vi "GEOM_AdjustDetStruct.vi"(7 "corr unbin":bool, 9 "GEOM_CorrectedFPA in":T1[](array[typedef]), 10 "GEOM_FPAReadModes":T2[](array[typedef]) {"Amplifiers"."fliped" items=["none", "horizontal", "vertical"]; "Amplifiers"."type" items=["LL", "LR", "UL", "UR"]}) -> ()   [LabVIEW 2016]
uses:
  GEOM_FPAReadMode.ctl
  GEOM_Amplifier.ctl
  GEOM_AmpType.ctl
  GEOM_ROI.ctl
  GEOM_Coords.ctl
  GEOM_CorrectedFPA.ctl
  GEOM_VAR_action.ctl
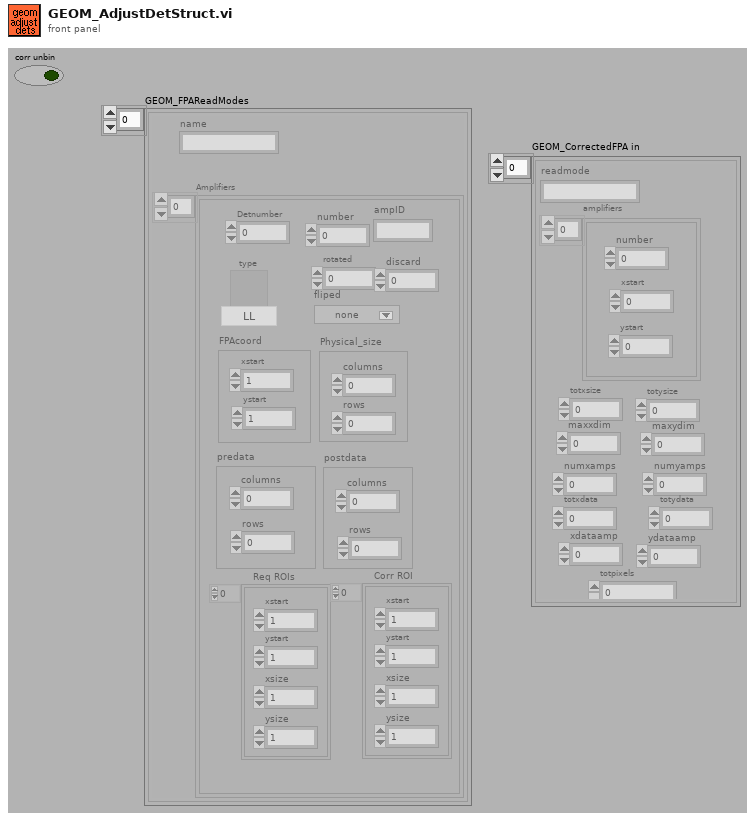
[diagram p1: front panel]
types:
  T1 = typedef "GEOM_CorrectedFPA.ctl" = cluster{"readmode":string, "amplifiers":cluster{"number":i32, "xstart":i32, "ystart":i32}[], "totxsize":i32, "totysize":i32, "maxxdim":i32, "maxydim":i32, "numxamps":i32, "numyamps":i32, "totxdata":i32, "totydata":i32, "xdataamp":i32, "ydataamp":i32, "totpixels":i32}
  T2 = typedef "GEOM_FPAReadMode.ctl" = cluster{"name":string, "Amplifiers":T3[]}
  T3 = typedef "GEOM_Amplifier.ctl" = cluster{"number":i32, "type":T4, "rotated":i16, "fliped":u16, "FPAcoord":cluster{"xstart":i32, "ystart":i32}, "Physical_size":cluster{"columns":i32, "rows":i32}, "predata":cluster{"columns":i32, "rows":i32}, "postdata":cluster{"columns":i32, "rows":i32}, "Req ROIs":T5, "Corr ROI":T5, "Detnumber":i32, "ampID":string, "discard":i32}
  T4 = typedef "GEOM_AmpType.ctl" = u16
  T5 = typedef "GEOM_ROI.ctl" = T6[]
  T6 = typedef "GEOM_Coords.ctl" = cluster{"xstart":u32, "ystart":u32, "xsize":u32, "ysize":u32}
  T7 = typedef "GEOM_VAR_action.ctl" = enum16{"read", "write"}
  T8 = typedef "GEOM_DetSummaryStruct.ctl" = cluster{"detxpos":i32, "detypos":i32, "cols":i32, "rows":i32, "nxamps":i32, "nyamps":i32, "number":i32, "discard":i32, "totcols":i32, "totrows":i32, "readmode":string}
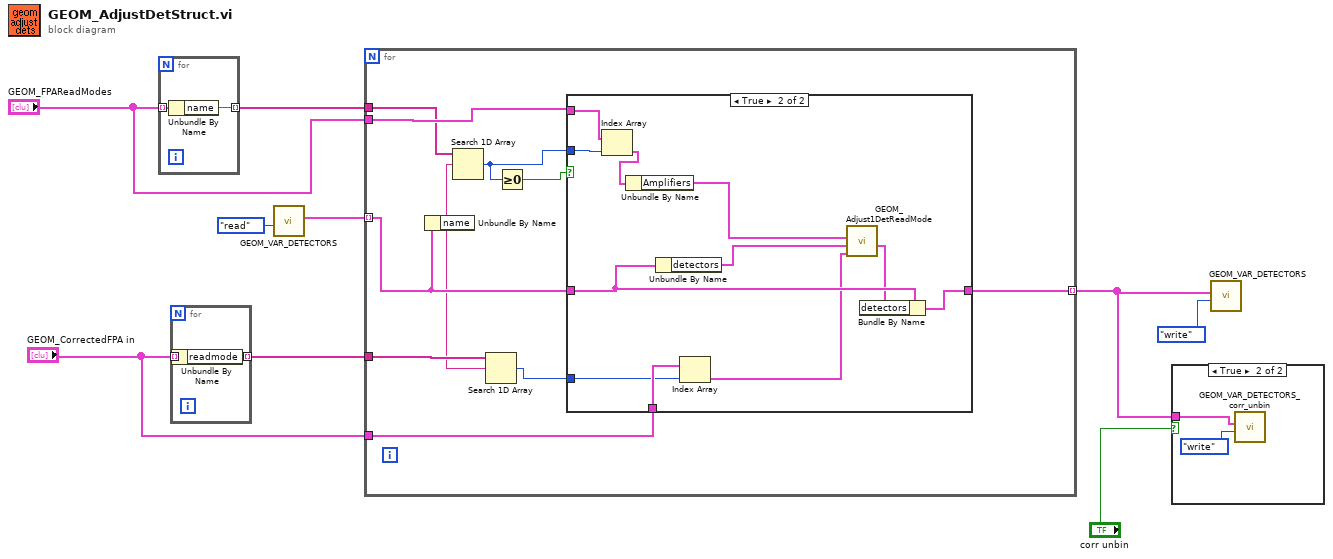
[diagram p0: block diagram]
diagram:
  n1 = for {
    tunnel: "GEOM_FPAReadModes" -> [w11] mode=indexing
    tunnel: [w10] -> w6 mode=indexing
    n2 = Unbundle By Name(w11) -> ("name"=w10:string)
  }
  n3 = for {
    tunnel: "GEOM_CorrectedFPA in" -> [w13] mode=indexing
    tunnel: [w12] -> w4 mode=indexing
    n4 = Unbundle By Name(w13) -> ("readmode"=w12:string)
  }
  n5 = call "GEOM_VAR_DETECTORS.vi"("Action"=GEOM_VAR_action."read") -> ("det out"=w8:cluster{"name":string, "detectors":T8[]}[])  [unwired: 1 in, 9 out]
  n6 = for {
    tunnel: "GEOM_FPAReadModes" -> [w23]
    tunnel: w8 -> [w21] mode=indexing
    tunnel: [w22] -> w2 mode=indexing
    tunnel: w6 -> [w20]
    tunnel: "GEOM_CorrectedFPA in" -> [w15]
    tunnel: w4 -> [w17]
    n7 = Unbundle By Name(w21) -> ("name"=w16:string)
    n8 = Search 1D Array(1D array=w20, element=w16) -> (index of element=w18:i32)  [unwired: 1 out]
    n9 = Search 1D Array(1D array=w17, element=w16) -> (index of element=w14:i32)  [unwired: 1 out]
    n10 = Greater Or Equal To 0?(x=w18) -> (x >= 0?=w19:bool)
    n11 = case shown="True" w19 {
      tunnel: w23 -> [_ w30]
      tunnel: [w24 w31] -> w22
      tunnel: w21 -> [w24 w33]
      tunnel: w18 -> [_ w29]
      tunnel: w15 -> [_ w27]
      tunnel: w14 -> [_ w26]
      frame False {
      }
      frame True {
        n12 = Index Array(array=w30, index=w29) -> (element=w28:T2)
        n13 = Unbundle By Name(w28) -> ("Amplifiers"=w35:T3[])
        n14 = Unbundle By Name(w33) -> ("detectors"=w34:T8[])
        n15 = Index Array(array=w27, index=w26) -> (element=w25:T1)
        n16 = call "GEOM_Adjust1DetReadMode.vi"("GEOM_BinCorrectedFPA"=w25, "detectors"=w34, "Amplifiers"=w35) -> ("detectors out"=w32:T8[])  [unwired: 8 out]
        n17 = Bundle By Name(cluster=w33, "detectors"=w32) -> (w31:cluster{"name":string, "detectors":T8[]})
      }
    }
  }
  n18 = case shown="True" "corr unbin" {
    tunnel: w2 -> [_ w36]
    frame False {
    }
    frame True {
      n19 = call "GEOM_VAR_DETECTORS_corr_unbin.vi"("Action"=GEOM_VAR_action."write", "det in"=w36) -> ()  [unwired: 10 out]
    }
  }
  n20 = call "GEOM_VAR_DETECTORS.vi"("Action"=GEOM_VAR_action."write", "det in"=w2) -> ()  [unwired: 10 out]
